vi "Set Sub Number.vi"(8 "error in":errorcluster, 10 "Sub Number":u8, 11 "Object Entry in":refnum<class "Object Entry.lvclass">) -> (0 "error out":errorcluster, 3 "Object Entry out":refnum<class "Object Entry.lvclass">)   [LabVIEW 2020, in "CANopen.lvlib" / "Object Entry.lvclass"]
uses:
  Object Entry.lvclass
  Object Entry.lvclass/Object Entry.ctl
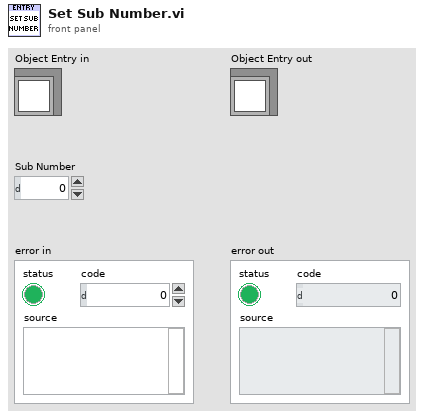
[diagram p1: front panel]
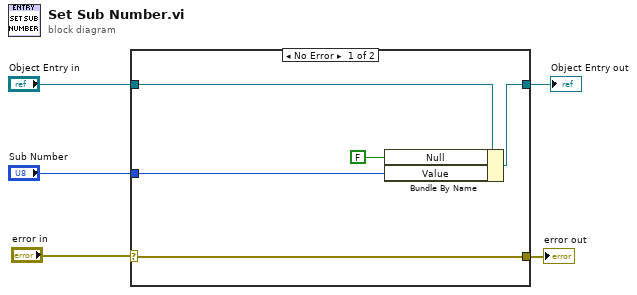
[diagram p0: block diagram]
diagram:
  n1 = case shown="No Error" "error in" {
    selector: "error in" -> [w10 w11]
    tunnel: [w10 w11] -> w2
    tunnel: [w8 w12] -> w4
    tunnel: "Object Entry in" -> [w9 w12]
    tunnel: "Sub Number" -> [w7 _]
    frame No Error {
      n2 = Bundle By Name(cluster=w9, "Null"=FALSE ("Sub Number.Null"), "Value"=w7) -> (w8:refnum<class "Object Entry.lvclass">)
    }
    frame Error {
    }
  }
  "error out" <- w2
  "Object Entry out" <- w4
